vi "I2C Write.vi"(5 "EOF":T1, 7 "I2C Channel":u8, 8 "Error In":errorcluster, 9 "Data":u8[](array[numeric])=[0], 10 "I2C Slave Address (0)":u8, 11 "LINX Resource":T2={"IO"=enum."Remote", "Interface"=enum."TCP", "LINX Device Config"={"Interface"=enum."TCP", "COM Port"="N/A", "TCP Configuration"={"IP Address"="panicattack", "Port"=6999}, "Device Family"=4, "Device ID"=1, "Device Name"="Raspberry Pi Model B", "TCP Ref"=refnum, "Channels"={"DI"=[2, 3, 4, 7, 8, 9, 10, 11, 14, 15, 17, 18, 22, 23, 24, 25, 27], "DO"=[2, 3, 4, 7, 8, 9, 10, 11, 14, 15, 17, 18, 22, 23, 24, 25, 27], "AI"=[], "AO"=[], "PWM"=[], "QE"=[], "UART"=[0], "I2C 2"=[0, 1], "SPI"=[0], "CAN"=[], "Servo"=[], "AI Ref (V)"=0.0, "AI Resolution (Bits)"=0, "AO Ref (V)"=0.0, "AO Resolution (Bits)"=0}}}) -> (0 "Error Out":errorcluster, 3 "LINX Resource":T2={"IO"=enum."Remote", "Interface"=enum."TCP", "LINX Device Config"={"Interface"=enum."TCP", "COM Port"="N/A", "TCP Configuration"={"IP Address"="panicattack", "Port"=6999}, "Device Family"=4, "Device ID"=1, "Device Name"="Raspberry Pi Model B", "TCP Ref"=refnum, "Channels"={"DI"=[2, 3, 4, 7, 8, 9, 10, 11, 14, 15, 17, 18, 22, 23, 24, 25, 27], "DO"=[2, 3, 4, 7, 8, 9, 10, 11, 14, 15, 17, 18, 22, 23, 24, 25, 27], "AI"=[], "AO"=[], "PWM"=[], "QE"=[], "UART"=[0], "I2C 2"=[0, 1], "SPI"=[0], "CAN"=[], "Servo"=[], "AI Ref (V)"=0.0, "AI Resolution (Bits)"=0, "AO Ref (V)"=0.0, "AO Resolution (Bits)"=0}}})   [LabVIEW 2020, in "LMH-LINX.lvlib"]
doc: "Write data bytes to the I2C slave device identified by I2C Slave Address on the specified I2C channel."
uses:
  LMH-LINX.lvlib
  Private/Type Defs/LINX Ref.ctl
  Private/Type Defs/Platform.ctl
  Private/Type Defs/Interface.ctl
  Private/Device/Type Defs/LINX Device Config.ctl
  Private/Device/Type Defs/TCP Config.ctl
  Private/Device/Type Defs/Channels.ctl
  Private/Type Defs/Peripherals/I2C/EOF.ctl
  Private/Type Defs/Peripheral.ctl
  Private/Utilties/Generate Error.vi
  Private/Device/Device.lvlib
  Private/Local IO/Local IO.lvlib
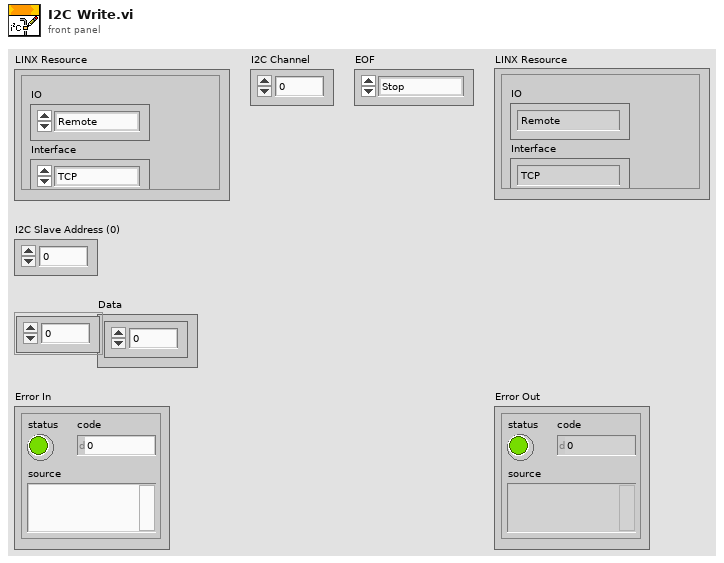
[diagram p1: front panel]
types:
  T1 = typedef "LMH-LINX.lvlib/EOF.ctl" = enum8{"Stop", "Restart", "Restart No Stop", "No Stop"}
  T2 = typedef "LMH-LINX.lvlib/LINX Ref.ctl" = cluster{"IO":T3, "Interface":T4, "LINX Device Config":T5}
  T3 = typedef "LMH-LINX.lvlib/Platform.ctl" = enum16{"Remote", "Local"}
  T4 = typedef "LMH-LINX.lvlib/Interface.ctl" = enum16{"Serial", "TCP"}
  T5 = typedef "LMH-LINX.lvlib/Device.lvlib/LINX Device Config.ctl" = cluster{"Interface":T4, "COM Port":refnum<visa-resource-name>, "TCP Configuration":T6, "Device Family":u8, "Device ID":u8, "Device Name":string, "TCP Ref":refnum<k5>, "Channels":T7}
  T6 = typedef "LMH-LINX.lvlib/Device.lvlib/TCP Config.ctl" = cluster{"IP Address":string, "Port":u16}
  T7 = typedef "LMH-LINX.lvlib/Channels.ctl" = cluster{"DI":u8[], "DO":u8[], "AI":u8[], "AO":u8[], "PWM":u8[], "QE":u8[], "UART":u8[], "I2C 2":u8[], "SPI":u8[], "CAN":u8[], "Servo":u8[], "AI Ref (V)":dbl, "AI Resolution (Bits)":u8, "AO Ref (V)":dbl, "AO Resolution (Bits)":u8}
  T8 = typedef "LMH-LINX.lvlib/Peripheral.ctl" = enum8{"DI", "DO", "AI", "AO", "PWM", "QE", "UART", "I2C", "SPI", "CAN", "Servo"}
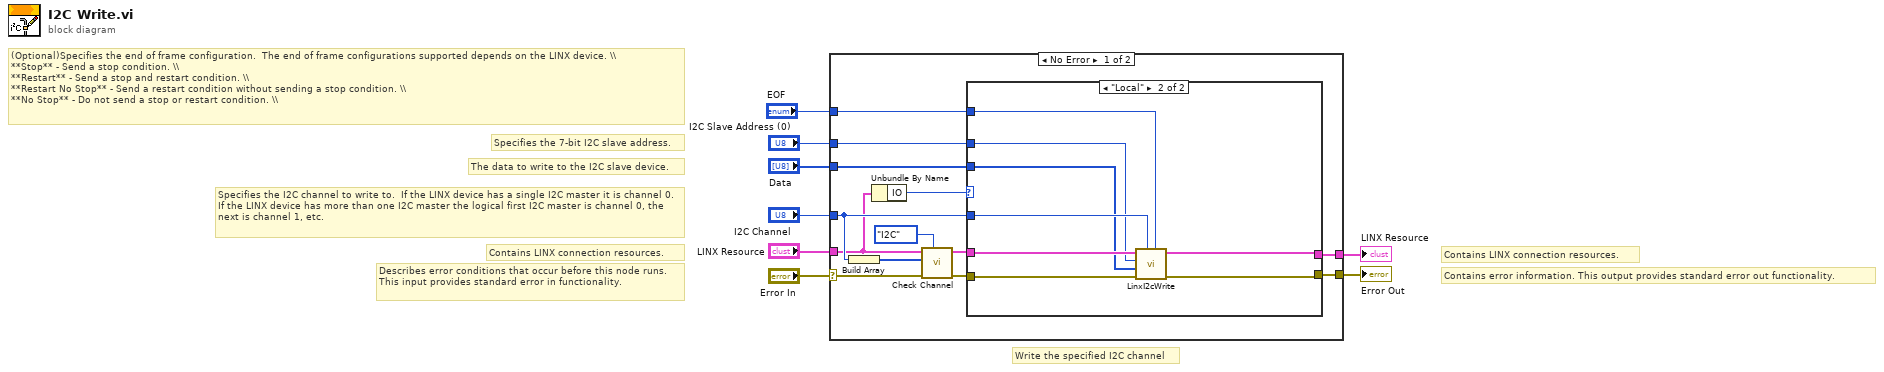
[diagram p0: block diagram]
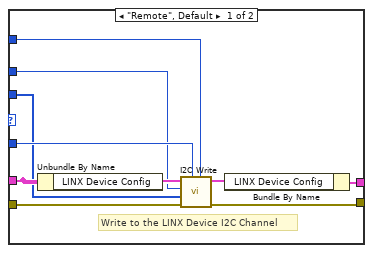
[diagram p2: hidden frame]
diagram:
  # "The data to write to the I2C slave device."
  # "Specifies the 7-bit I2C slave address."
  # "(Optional)Specifies the end of frame configuration.  The end of frame configurations supported depends on the LINX device. \\\\ \n**Stop** - Send a stop condition. \\\\ \n**Restart** - Send a stop and restart condition. \\\\\n**Restart No Stop** - Send a restart condition without sending a stop condition. \\\\ \n**No Stop** - Do not send a stop or restart condition. \\\\"
  # "Specifies the I2C channel to write to.  If the LINX device has a single I2C master it is channel 0.  If the LINX device has more than one I2C master the logical first I2C master is channel 0, the next is channel 1, etc."
  # "Contains LINX connection resources."
  # "Contains error information. This output provides standard error out functionality."
  # "Contains LINX connection resources."
  # "Describes error conditions that occur before this node runs. This input provides standard error in functionality."
  # "Write the specified I2C channel"
  n1 = case shown="No Error" "Error In" {
    selector: "Error In" -> [w9 w41]
    tunnel: [w20 w41] -> w8
    tunnel: [w19 w40] -> w7
    tunnel: "Data" -> [w18 _]
    tunnel: "I2C Slave Address (0)" -> [w17 _]
    tunnel: "I2C Channel" -> [w14 _]
    tunnel: "LINX Resource" -> [w12 w40]
    tunnel: "EOF" -> [w10 _]
    frame No Error {
      n2 = Build Array(w14) -> (w13:u8[])
      n3 = Unbundle By Name(w12) -> ("IO"=w21:T3)
      n4 = call "Check Channel.vi"("Peripheral"=Peripheral."I2C", "Error In"=w9, "Channels"=w13, "LINX Resource"=w12) -> ("Error Out"=w15:errorcluster, "LINX Resource"=w11:T2)  [unwired: 5 in, 1 out]
      n5 = case shown="\"Local\"" w21 {
        tunnel: w15 -> [w28 w36]
        tunnel: w11 -> [w31 w39]
        tunnel: [w29 w37] -> w20
        tunnel: [w30 w38] -> w19
        tunnel: w14 -> [w25 w35]
        tunnel: w18 -> [w23 w32]
        tunnel: w17 -> [w24 w34]
        tunnel: w10 -> [w22 w33]
        frame "Remote", Default {
          # "Write to the LINX Device I2C Channel"
          n6 = Unbundle By Name(w31) -> ("LINX Device Config"=w26:T5)
          n7 = call "I2C Write.vi"("EOF"=w22, "I2C Channel (0)"=w25, "Error In"=w28, "Data"=w23, "I2C Slave Address"=w24, "LINX Device Config"=w26) -> ("Error Out"=w29:errorcluster, "LINX Device Config"=w27:T5)  [unwired: 4 in]
          n8 = Bundle By Name(cluster=w31, "LINX Device Config"=w27) -> (w30:T2)
        }
        frame "Local" {
          n9 = call "LinxI2cWrite.vi"("EOF"=w33, "I2C Channel"=w35, "Error In"=w36, "Data"=w32, "Slave Address"=w34, "LINX Resource"=w39) -> ("Error Out"=w37:errorcluster, "LINX Resource"=w38:T2)  [unwired: 4 in]
        }
      }
    }
    frame Error {
    }
  }
  "Error Out" <- w8
  "LINX Resource" <- w7
